vi "Set Do.vi"(8 "error in (no error)":errorcluster, 9 "Indx":i32, 10 "Value":bool, 11 "reference in":refnum<class "FPGA_Mock.lvclass">) -> (0 "error out":errorcluster, 3 "reference out":refnum<class "FPGA_Mock.lvclass">)   [LabVIEW 2019, in "FPGA_Mock.lvclass"]
uses:
  FPGA_Mock.lvclass
  FPGA_Mock.lvclass/FPGA_Mock.ctl
  b762c7e6-3419-48e6-af3f-ce84c66988ed.vi
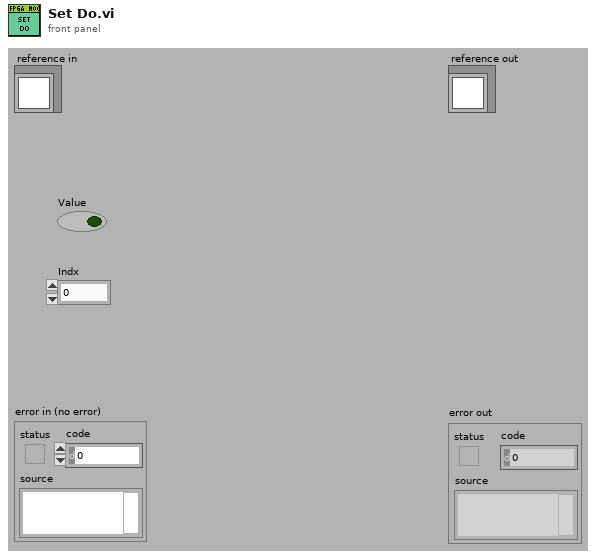
[diagram p1: front panel]
types:
  T1 = typedef "FPGA_Mock.lvclass/SharedData.ctl" = cluster{"DI":bool[], "DO":bool[], "AO":dbl[]}
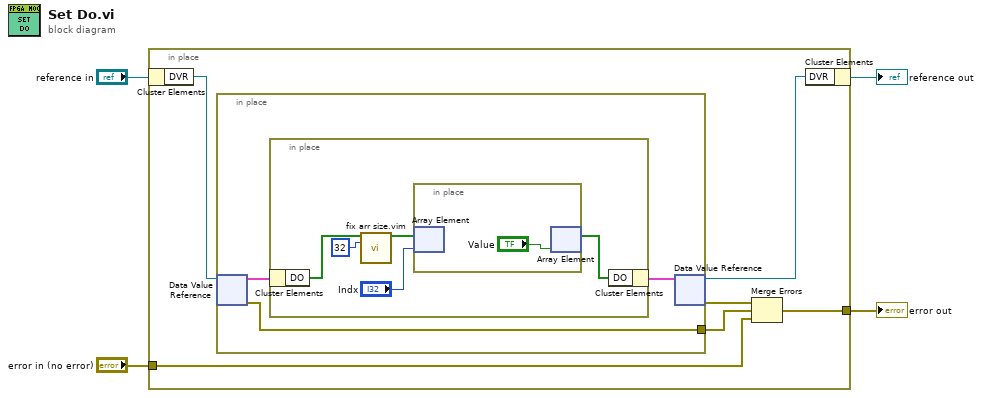
[diagram p0: block diagram]
diagram:
  n1 = in-place {
    in-place-border: "error in (no error)" -> [w5]
    in-place-border: [w6] -> w1
    n2 = in-place-cluster #1("reference in") -> ("DVR"=w10:refnum<data-value>)
    n3 = in-place {
      in-place-border: [w13] -> w8
      n4 = in-place-dvr #2(w10) -> (w12:T1, w13:errorcluster)
      n5 = in-place {
        n6 = in-place-cluster #3(w12) -> ("DO"=w16:bool[])
        n7 = call "fix arr size.vim"("arr in"=w16, "Size"=32) -> ("arr out"=w15:bool[])  [unwired: 13 in]
        n8 = in-place {
          n9 = in-place-array #4(w15, "Indx") -> ()  [unwired: 1 out]
          n10 = in-place-array #4("Value") -> (w18:bool[])  [unwired: 1 out]
        }
        n11 = in-place-cluster #3("DO"=w18) -> (w11:T1)
      }
      n12 = in-place-dvr #2(w11) -> (w9:refnum<data-value>, w7:errorcluster)
    }
    n13 = Merge Errors(w7, w8, w5) -> (w6:errorcluster)
    n14 = in-place-cluster #1("DVR"=w9) -> (→"reference out":refnum<class "FPGA_Mock.lvclass">)
  }
  "error out" <- w1
